vi "Voltage measurment on multimeter.vi"(8 "error in (no error)":errorcluster, 10 "Function (0: DC Volts) 2":u16(ring)=1 items=["DC Volts", "AC Volts", "DC Current", "AC Current", "2-Wire Resistance", "4-Wire Resistance"], 11 "VISA resource name 3":refnum<visa-resource-name>="USB0::0x1AB1::0x0C94::DM3O194400985::INSTR") -> (0 "error out":errorcluster, 3 "Digital Display":dbl)   [LabVIEW 2018]
uses:
  <instrlib>/RIGOL DM3058/RIGOL DM3058.lvlib
panel:
  in  "Absolute Resolution (0: 5.5 Rate:Slow)":u16(ring)=2 items=["5.5 Rate:Slow", "4.5 Rate:Middle", "4.5 Rate:Fast", "3.5 Rate", "6.5 Rate"]
  out "Gauge":dbl(knob) scale=0.0..150.0
  in  "Manual Range (1.0) 2":dbl=1.0
  in  "Auto Range (T: Enable) 2":bool=TRUE
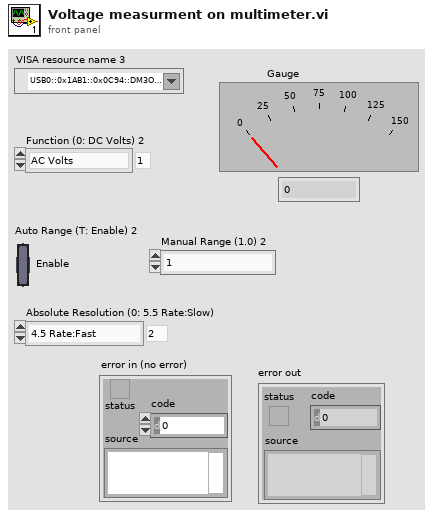
[diagram p1: front panel]
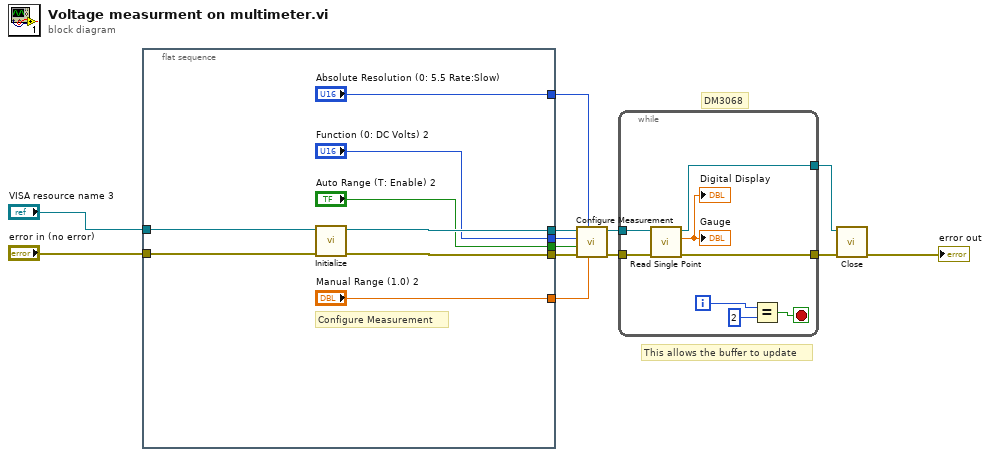
[diagram p0: block diagram]
diagram:
  # "This allows the buffer to update"
  # "DM3068"
  n1 = flat-sequence {
    tunnel: [w21] -> w7
    tunnel: [w20] -> w8
    tunnel: ["Function (0: DC Volts) 2"] -> w9
    tunnel: ["Manual Range (1.0) 2"] -> w10
    tunnel: ["Auto Range (T: Enable) 2"] -> w11
    tunnel: "VISA resource name 3" -> [w16]
    tunnel: "error in (no error)" -> [w15]
    tunnel: ["Absolute Resolution (0: 5.5 Rate:Slow)"] -> w1
    frame #0 {
      # "Configure Measurement"
      n2 = call <instrlib>:"Initialize.vi"("error in (no error)"=w15, "VISA resource name"=w16) -> ("error out"=w20:errorcluster, "VISA resource name out"=w21:refnum<visa-resource-name>)  [unwired: 3 in, 5 out]
    }
  }
  n3 = call <instrlib>:"Configure Measurement.vi"("Manual Range (1.00)"=w10, "Absolute Resolution (0: 5.5 Rate:Slow)"=w1, "error in (no error)"=w8, "Auto Range (T:Enable)"=w11, "Function (0: DC Volts)"=w9, "VISA resource name"=w7) -> ("error out"=w12:errorcluster, "VISA resource name out"=w13:refnum<visa-resource-name>)  [unwired: 4 out]
  n4 = while {
    tunnel: w13 -> [w29]
    tunnel: [w27] -> w5
    tunnel: w12 -> [w28]
    tunnel: [w26] -> w6
    i -> [w22]
    stop <- w24 stop-if-true
    n5 = call <instrlib>:"Read Single Point.vi"("error in (no error)"=w28, "VISA resource name"=w29) -> ("error out"=w26:errorcluster, "Measurement"=→"Gauge" →"Digital Display":dbl, "VISA resource name out"=w27:refnum<visa-resource-name>)  [unwired: 7 out]
    n6 = Equal?(x=w22, y=u32 2) -> (x = y?=w24:bool)
  }
  n7 = call <instrlib>:"Close.vi"("error in (no error)"=w6, "VISA resource name"=w5) -> ("error out"=→"error out":errorcluster)  [unwired: 9 out]
